vi "Test Math Operations.vi"() -> ()   [LabVIEW 2026]
doc: "Test Math Ops"
panel:
  out "XY Graph":cluster{dbl[], dbl[]}(graph)
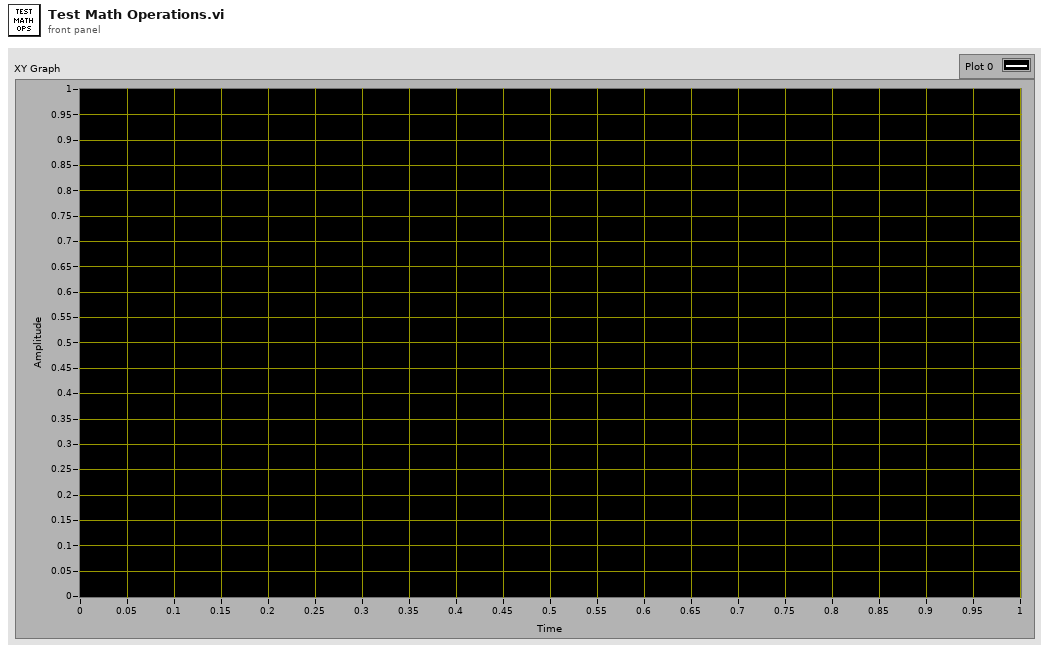
[diagram p1: front panel]
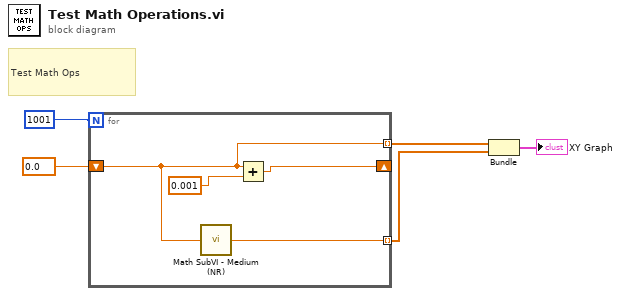
[diagram p0: block diagram]
diagram:
  # "Test Math Ops"
  n1 = for {
    N: 1001 -> [_]
    shift-right: [w7] -> _
    shift-left: 0.0 -> [w6]
    tunnel: [w9] -> w2 mode=indexing
    tunnel: [w6] -> w3 mode=indexing
    n2 = call "Math SubVI - Medium (NR).vi"("Input"=w6) -> ("Output"=w9:dbl)
    n3 = Add(x=w6, y=0.001) -> (x+y=w7:dbl)
  }
  n4 = Bundle(w3, w2) -> (→"XY Graph":cluster{dbl[], dbl[]})  [unwired: 1 in]
